vi "IV.vi"(2 "Run uninterrupted?":bool, 3 "Device Category IN:":string(combo)="ATLAS18SS" caption="Device Category:", 4 "Batch No. IN:":string caption="Batch No.:", 5 "Wafer No. IN:":string caption="Wafer No.:", 6 "DB Serial No. IN:":string caption="DB Serial No.:") -> (0 "Done!":bool)   [LabVIEW 2013]
doc: "Performs IV measurements according to ATLAS ITk Quality Control Specifications."
uses:
  InstrControl/Switching/Switching.lvclass
  InstrControl/SupplyControl/SupplyControl.lvclass
  general_VIs/globals/QC_MeasurementSetup.vi
  general_VIs/globals/QC_RunInformation.vi
  InstrControl/InstrumentSetup.vi
  InstrControl/ArduinoControl/ArduinoControl.lvclass
  <vilib>/Analysis/NI_AALBase.lvlib
  InstrControl/InstrControl.lvclass
panel:
  out "Tab Control 2":enum32{"IV Setup", "IV Scan"}(tab)
  in  "V_breakdown limit [V]":dbl=-500.0
  in  "Set current limit?":bool
  in  "Current Limit [µA]":dbl=1000.0 min=0.0001 format="%.3f"
  in  "Measurement Configurations":bool
  in  "hold steps IN":i32=6 caption="hold steps"
  in  "Initial volts [V] IN":dbl caption="Initial volts [V]"
  in  "Final volts [V] IN":dbl=-700.0 caption="Final volts [V]"
  in  "step [V] IN":dbl=10.0 caption="step [V]" format="%.1f"
  in  "step interval [s] IN":i32=10 caption="step interval [s]"
  in  "Continue":bool
  in  "Quit":bool
  out "hold steps":i32=6
  out "RH":dbl[](array[numeric]) caption="RH [%]" format="%#.2f"
  out "Temp.":dbl[](array[numeric]) caption="Temp. [°C]" format="%#.2f"
  out "Current":dbl[](array[numeric]) caption="Current [nA]"
  out "Volts":dbl[](array[numeric]) caption="Volts [V]"
  out "step interval [s]":i32=10
  out "step [V]":dbl=10.0 format="%.1f"
  out "Final volts [V]":dbl=-700.0 format="%.1f"
  out "Initial volts [V]":dbl format="%.1f"
  out "Igraph":cluster{dbl[], dbl[]}(graph)
  in  "Scales":T1(ring)
  in  "Iscale":enum16{"nanoAmps", "microAmps", "milliAmps"}(ring)
  out "positive ramp?":bool
  out "Tab Control":enum32{"IV Setup", "IV Scan"}(tab)
  in  "Hardware Configurations":bool
  in  "User:":string(combo)="Christoph"
  in  "IV Supply":string(combo)="Keithley 2410"
  in  "Temperature":enum16{"Read Arduino", "Enter manually"}(ring)
  in  "Manufacturer:":string(combo)="Hamamatsu"
  in  "abort":bool
  out "Device Category:":string
  out "DB Serial No.:":string
  out "Current Volts:":dbl format="%.2f"
  in  "quit (no save)":bool
  in  "Quit & Save":bool
  out "Bias On/Off:":bool
  out "STATUS 1":string
  out "Initiated:":string
  out "Sensor No.:":string
  out "No of steps":u32
  out "Current reading No.":u32
  out "Last reading at:":string
  # "University of\nCambridge"
  # "Strip Sensor QC: IV"
  # "Vertical Scale:"
  # "Measurement Configuration"
  # "IV Scan parameters:"
  # "Last 5 readings:"
  # "n-4"
  # "n-3"
  # "n-2"
  # "n-1"
  # "n"
  # "DUT Description"
  # "Hardware"
  # "DUT & Test Description:"
  # "Current status:"
  # "Rdg No:"
  # "out of"
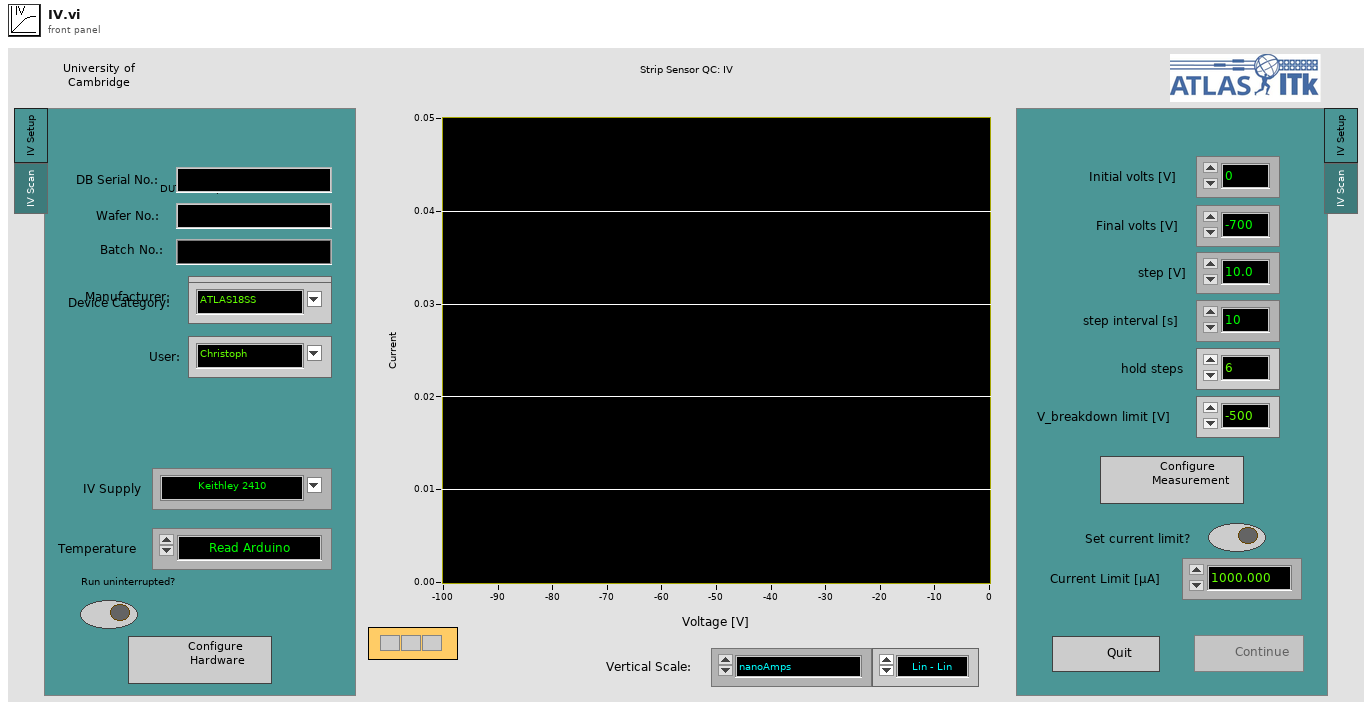
[diagram p1: front panel]
types:
  T1 = enum16{"Lin - Lin", "Log - Lin", "Lin - Log", "Log - log"}
  T2 = enum16{"Supply", "LCR", "Multimeter", "Switching"}
  T3 = enum16{"Reset", "Read Array", "Read Element", "Write Element", "Write Array", "Add Element", "Add Array"}
  T4 = enum16{"Reset", "Ground", "Striptest SMU", "Striptest LCR", "IV", "CV", "Interstrip Cap", "Interstrip Res"}
  T5 = enum32{"IV", "CV", "Stability", "Striptest", "Cis", "Ris", "PTP"}
  T6 = cluster{"Institute":string, "Manufacturers":string[], "Devices":string[], "Serialnumbers Lookup DB":string, "Data directory":string, "Backup & screenshot directory":string, "List of known users":string[], "Measurement switch not used":bool, "Measurement Switch":string, "DUT Switch":string, "Rseries IV [MOhm]":string, "Rshunt IV [MOhm]":string, "Rseries CV [MOhm]":string, "DC blocking Cap [µF]":string, "Rseries LCR [MOhm]":string, "Rseries stability [MOhm]":string, "Rshunt stability [MOhm]":string, "Rseries striptest bias [MOhm]":string, "Rseries strip pinhole [MOhm]":string}
  T7 = cluster{"Sensor Serial No.:":string, "Wafer:":string, "Batch:":string, "Manufacturer:":string, "Device Category:":string, "Database Serial No.:":string, "Date Initiated:":string, "Time Initiated:":string, "Test":string, "Probeplan used:":string, "End of Run comment:":string, "User:":string, "Vbias SMU":string, "LCR":string, "Test SMU":string, "Test DMM":string}
  T8 = cluster{"Supply":refnum<class "SupplyControl.lvclass">, "Arduino":refnum<class "ArduinoControl.lvclass">, "Measurement switch":refnum<class "Switching.lvclass">, "Initial Voltage [V]":dbl, "Final Voltage [V]":dbl, "Step Size [V]":dbl, "Step Interval [s]":i32, "Number Of Steps":u32, "Ramp down steps [V]":dbl, "Ramp down Interval [s]":i32, "hold steps":i32, "Set Current Limit?":bool, "Current Limit [µA]":dbl, "Temperature Readout":enum16{"Read Arduino", "Enter manually"}, "Supply Name":string, "V_breakdown Limit [V]":dbl, "Measurement switch used?":bool}
  T9 = cluster{"VISA address":refnum<visa-resource-name>, "T sensor":enum16{"SHT", "DS"}, "Arduino":refnum<class "ArduinoControl.lvclass">}
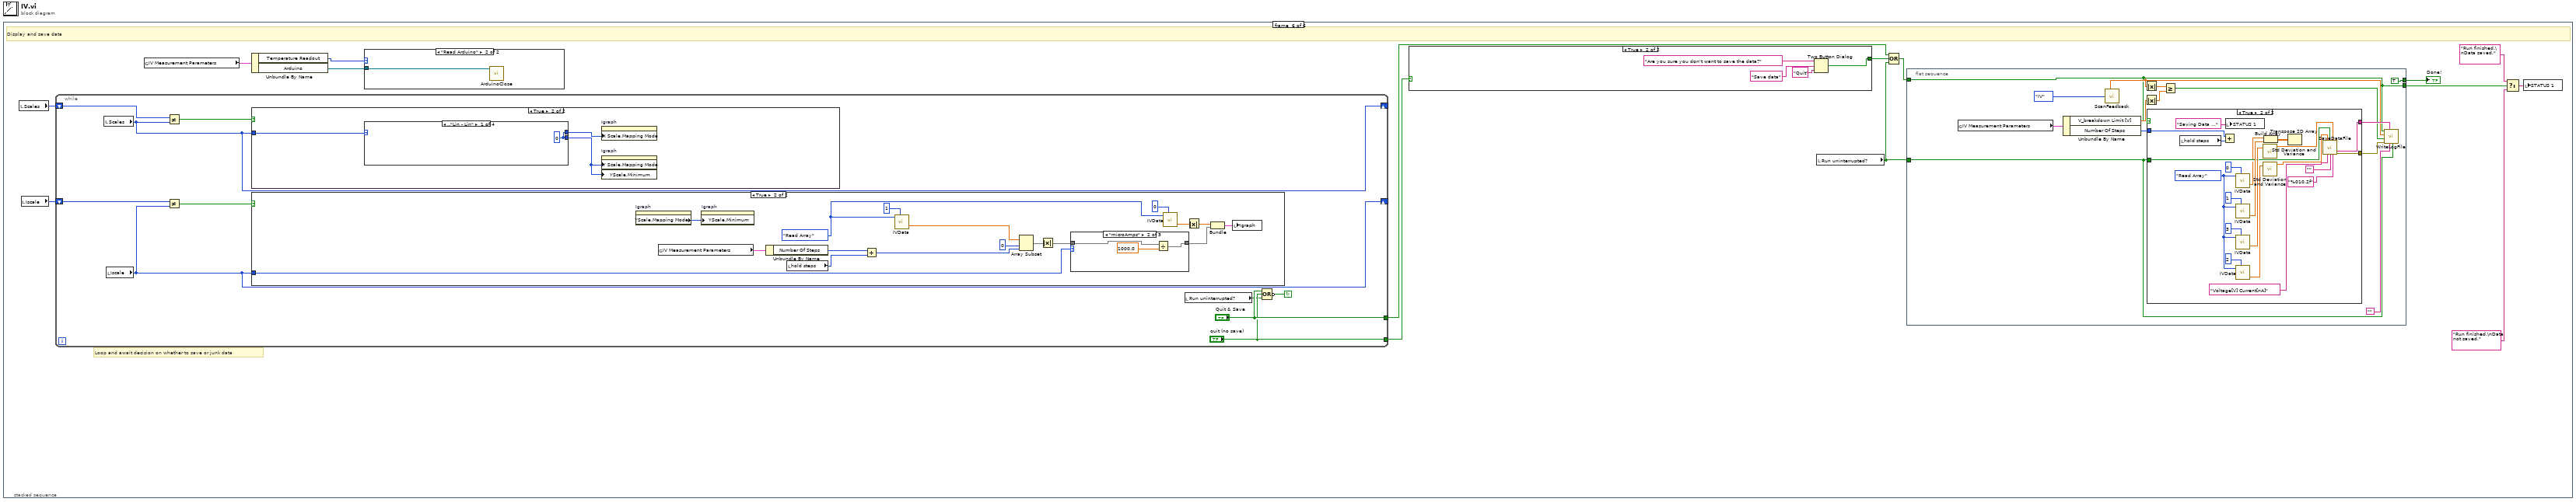
[diagram p0: block diagram]
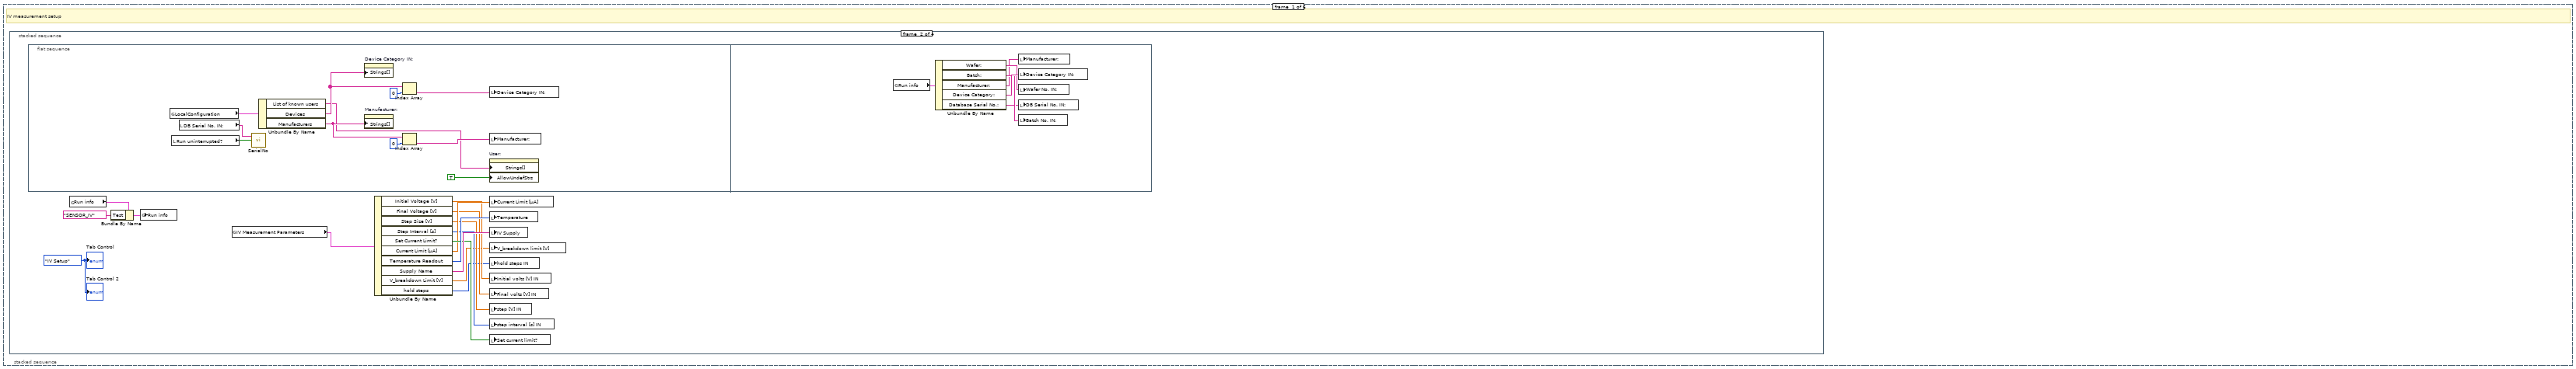
[diagram p2: hidden frame]
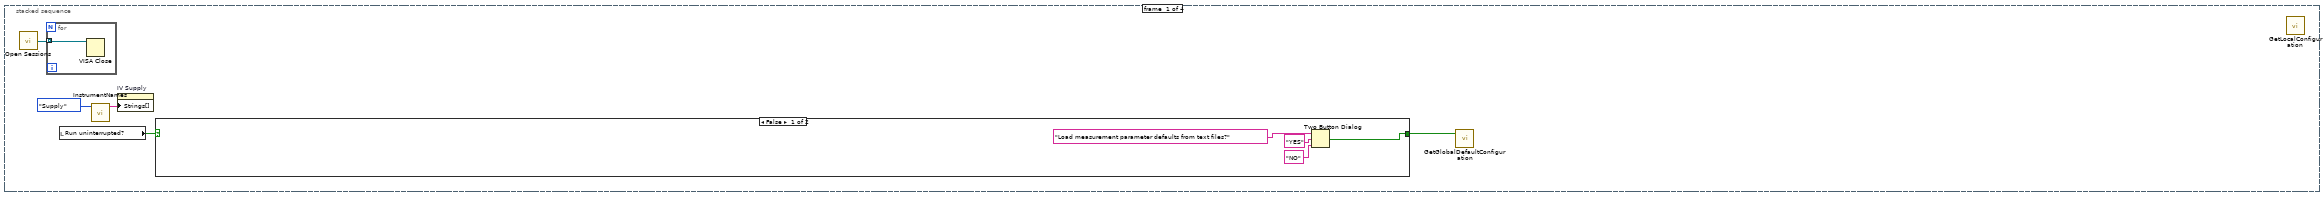
[diagram p3: hidden frame]
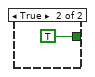
[diagram p4: hidden frame]
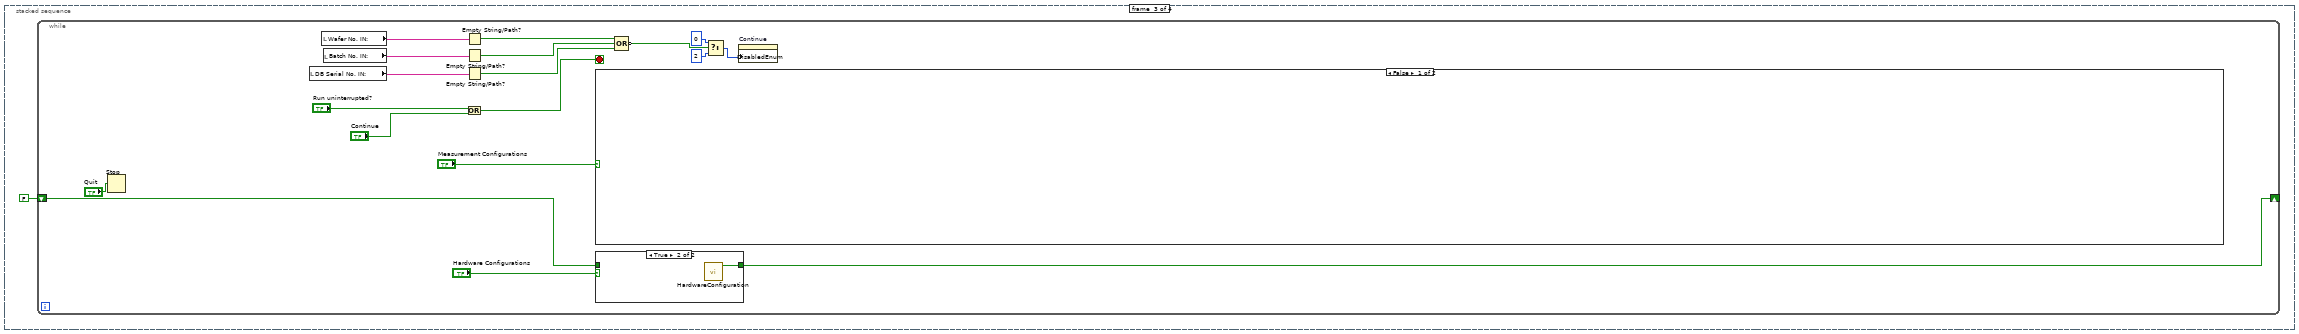
[diagram p5: hidden frame]
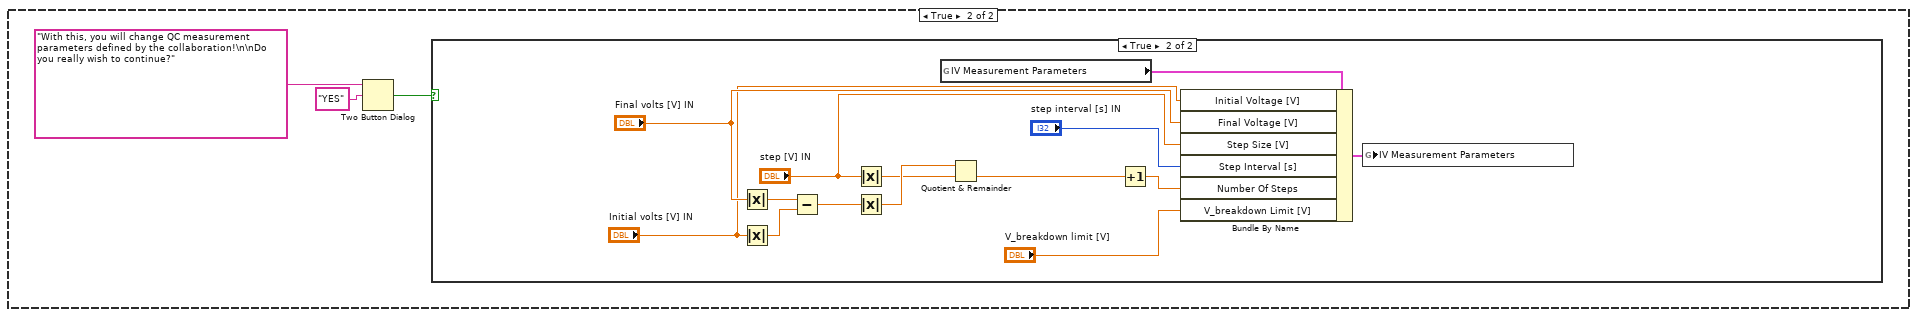
[diagram p6: hidden frame]
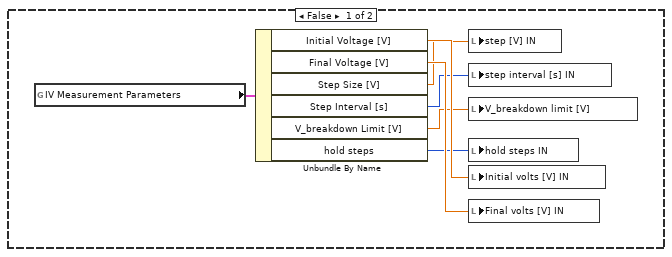
[diagram p7: hidden frame]
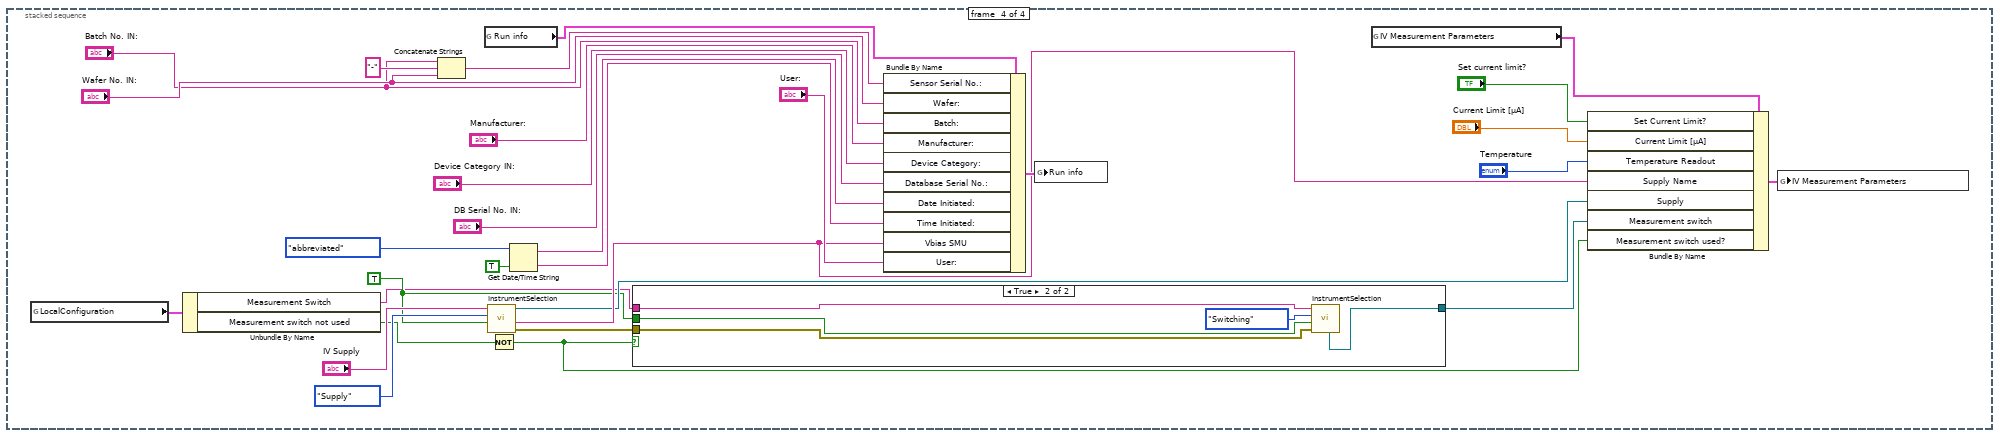
[diagram p9: hidden frame]
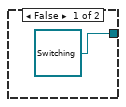
[diagram p10: hidden frame]
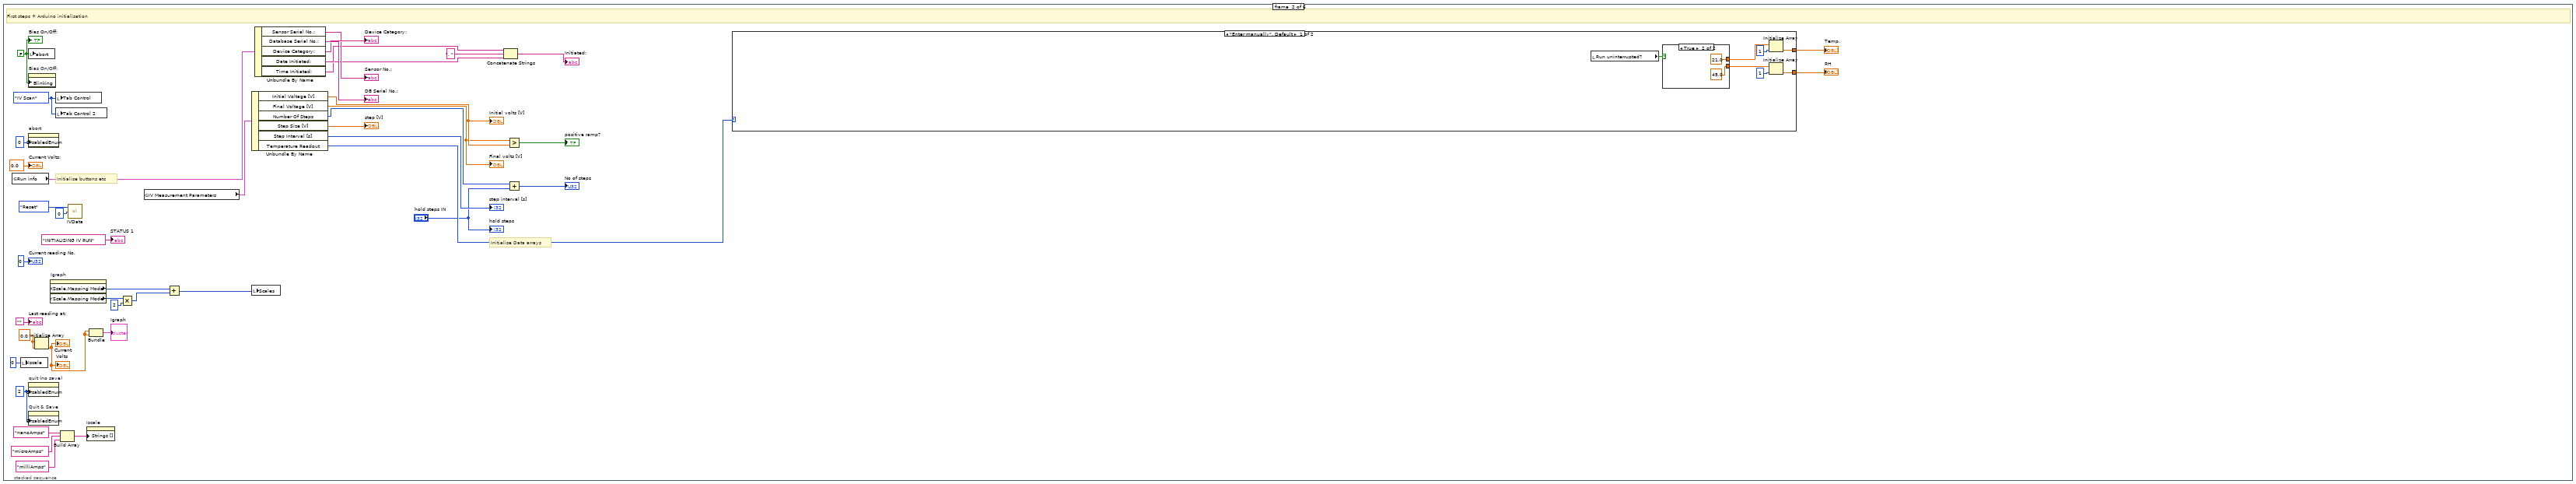
[diagram p11: hidden frame]
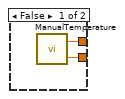
[diagram p12: hidden frame]
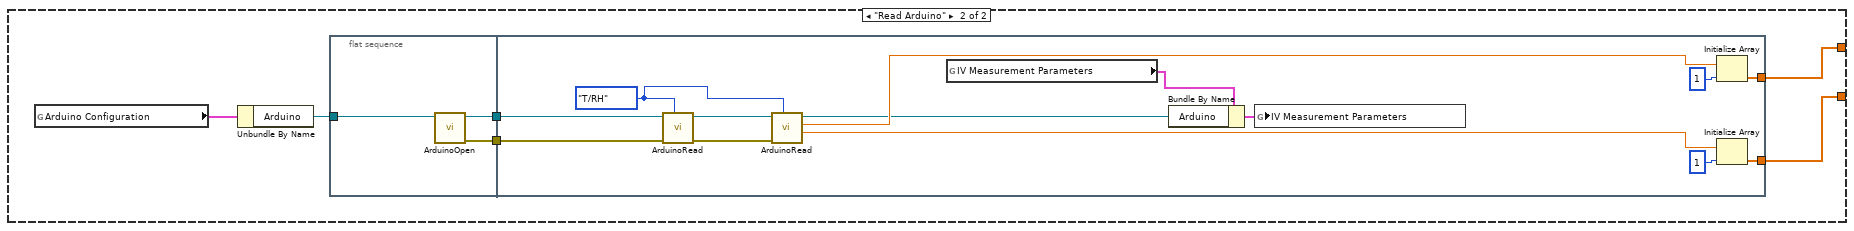
[diagram p13: hidden frame]
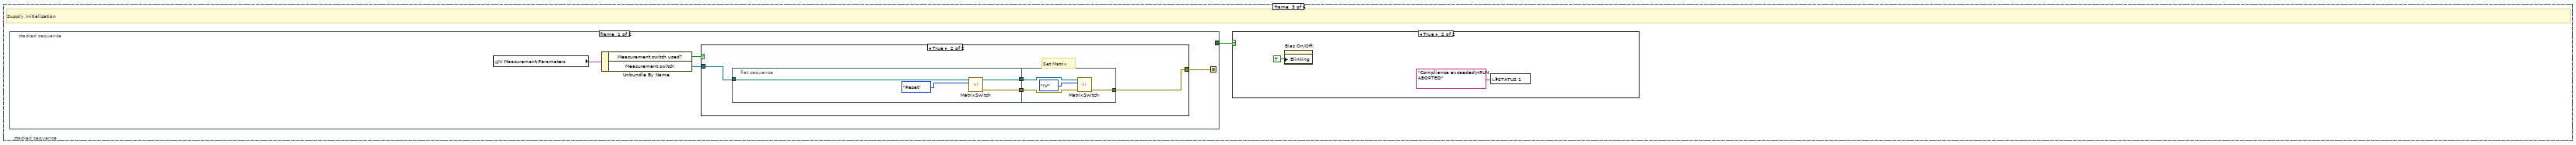
[diagram p14: hidden frame]
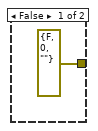
[diagram p15: hidden frame]
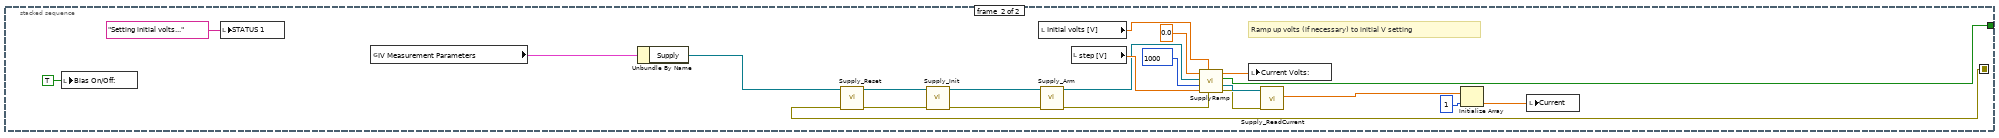
[diagram p16: hidden frame]
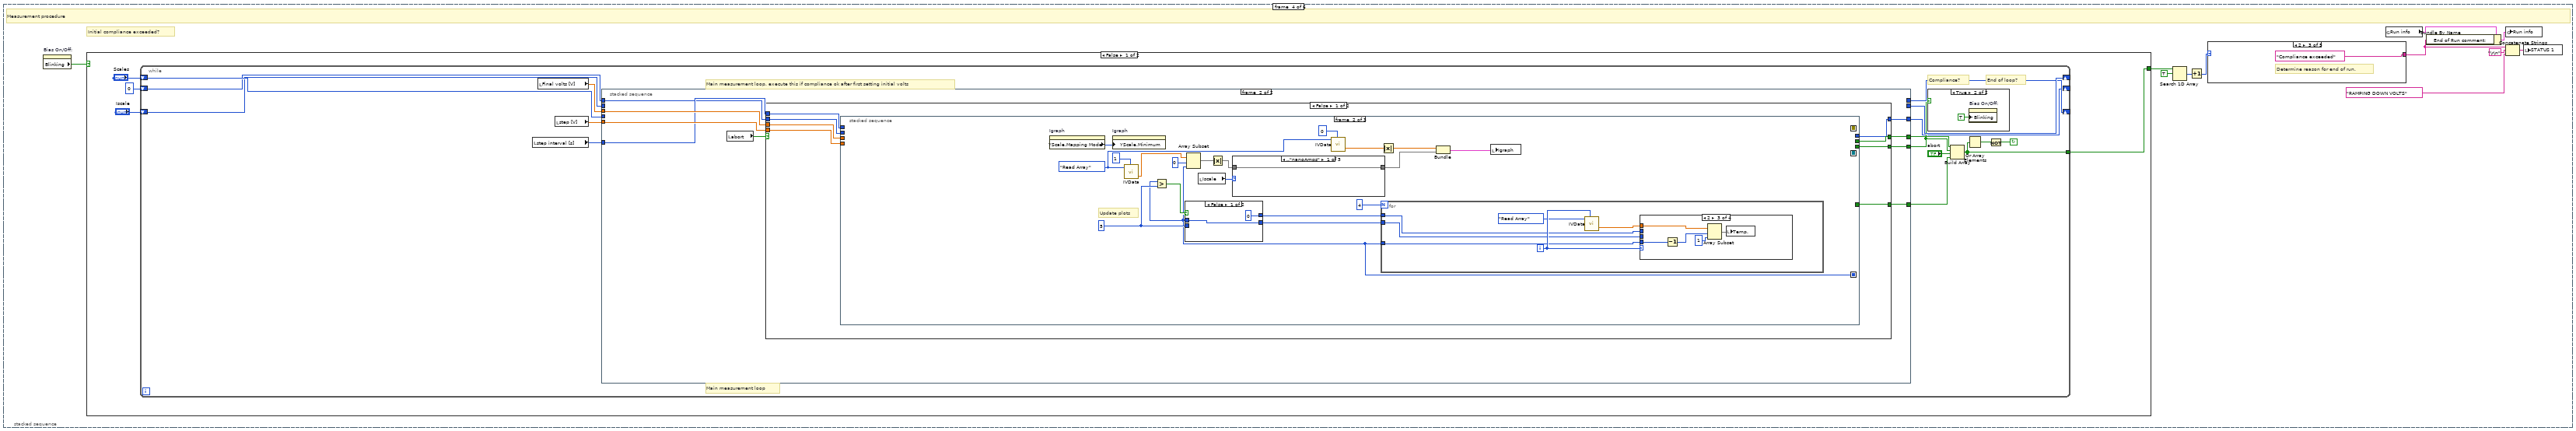
[diagram p18: hidden frame]
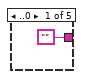
[diagram p19: hidden frame]
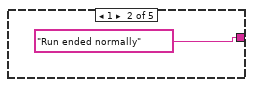
[diagram p20: hidden frame]
diagram:
  n1 = stacked-sequence {
    frame #0 {
      # "IV measurement setup"
      n2 = stacked-sequence {
        frame #0 {
          n3 = call <vilib>:"Open Sessions.vi"() -> ("Array of Refnums"=w1:refnum<visa-resource-name>[])  [unwired: 2 in]
          n4 = for {
            tunnel: w1 -> [w6] mode=indexing
            n5 = VISA Close(VISA resource name=w6) -> ()  [unwired: 1 in, 1 out]
          }
          n6 = local read "Run uninterrupted?"() -> (w2:bool)
          n7 = call "InstrumentNames.vi"("Instrument type"=T2."Supply") -> ("Instrument names"=w4:string[])  [unwired: 9 in, 1 out]
          n8 = property on="IV Supply" class="CmbBox"("Strings[]"=w4) -> ()  [unwired: 2 in, 2 out]
          n9 = case shown="False" w2 {
            tunnel: [w9 TRUE] -> w3
            frame False {
              n10 = Two Button Dialog(message="Load measurement parameter defaults from text files?", 1:"NO", 2:"YES") -> (T button?=w9:bool)
            }
            frame True {
            }
          }
          n11 = call "GetGlobalDefaultConfiguration.vi"("Read defaults?"=w3) -> ()  [unwired: 3 in]
          n12 = call "GetLocalConfiguration.vi"() -> ()  [unwired: 3 in, 1 out]
        }
        frame #1 {
          w19 = enum32{"IV Setup", "IV Scan"}."IV Setup" ("Tab Control")
          n13 = flat-sequence {
            frame #0 {
              n14 = global read "QC_RunInformation.vi" "LocalConfiguration"() -> (w29:T6)
              n15 = local read "Run uninterrupted?"() -> (w28:bool)
              n16 = local read "DB Serial No. IN:"() -> (w27:string)
              n17 = call "SerialNo.vi"("DB serial number IN"=w27, "Run uninterrupted?"=w28) -> ()  [unwired: 6 in, 2 out]
              n18 = Unbundle By Name(w29) -> ("List of known users"=w30:string[], "Devices"=w33:string[], "Manufacturers"=w35:string[])
              n19 = property on="Device Category IN:" class="CmbBox"("Strings[]"=w33) -> ()  [unwired: 2 in, 2 out]
              n20 = property on="Manufacturer:" class="CmbBox"("Strings[]"=w35) -> ()  [unwired: 2 in, 2 out]
              n21 = Index Array(array=w33, index=0) -> (element=w37:string)
              n22 = Index Array(array=w35, index=0) -> (element=w36:string)
              n23 = local write "Device Category IN:"(w37) -> ()
              n24 = local write "Manufacturer:"(w36) -> ()
              n25 = property on="User:" class="CmbBox"("Strings[]"=w30, "AllowUndefStrs"=TRUE) -> ()  [unwired: 2 in, 2 out]
            }
            frame #1 {
              n26 = global read "QC_RunInformation.vi" "Run info"() -> (w38:T7)
              n27 = Unbundle By Name(w38) -> ("Wafer:"=w42:string, "Batch:"=w41:string, "Manufacturer:"=w40:string, "Device Category:"=w43:string, "Database Serial No.:"=w39:string)
              n28 = local write "Manufacturer:"(w40) -> ()
              n29 = local write "Device Category IN:"(w43) -> ()
              n30 = local write "Wafer No. IN:"(w42) -> ()
              n31 = local write "DB Serial No. IN:"(w39) -> ()
              n32 = local write "Batch No. IN:"(w41) -> ()
            }
          }
          n33 = global read "QC_RunInformation.vi" "Run info"() -> (w21:T7)
          n34 = Bundle By Name(cluster=w21, "Test"="SENSOR_IV") -> (w20:T7)
          n35 = global write "QC_RunInformation.vi" "Run info"(w20) -> ()
          n36 = global read "QC_MeasurementSetup.vi" "IV Measurement Parameters"() -> (w24:T8)
          n37 = Unbundle By Name(w24) -> ("Initial Voltage [V]"=w17:dbl, "Final Voltage [V]"=w16:dbl, "Step Size [V]"=w15:dbl, "Step Interval [s]"=w18:i32, "Set Current Limit?"=w23:bool, "Current Limit [µA]"=w22:dbl, "Temperature Readout"=w26:enum16{"Read Arduino", "Enter manually"}, "Supply Name"=w25:string, "V_breakdown Limit [V]"=w14:dbl, "hold steps"=w13:i32)
          n38 = local write "Current Limit [µA]"(w22) -> ()
          n39 = local write "Temperature"(w26) -> ()
          n40 = local write "IV Supply"(w25) -> ()
          n41 = local write "V_breakdown limit [V]"(w14) -> ()
          n42 = local write "hold steps IN"(w13) -> ()
          n43 = local write "Initial volts [V] IN"(w17) -> ()
          n44 = local write "Final volts [V] IN"(w16) -> ()
          n45 = local write "step [V] IN"(w15) -> ()
          n46 = local write "step interval [s] IN"(w18) -> ()
          n47 = local write "Set current limit?"(w23) -> ()
          "Tab Control" <- w19
          "Tab Control 2" <- w19
        }
        frame #2 {
          n48 = while {
            shift-right: [w52] -> _
            shift-left: FALSE -> [w51]
            stop <- w48 stop-if-true
            n49 = Stop(stop? (T)="Quit") -> ()
            n50 = local read "DB Serial No. IN:"() -> (w46:string)
            n51 = local read "Wafer No. IN:"() -> (w61:string)
            n52 = local read "Batch No. IN:"() -> (w54:string)
            n53 = Empty String/Path?(string/path=w61) -> (empty?=w60:bool)
            n54 = Empty String/Path?(string/path=w54) -> (empty?=w53:bool)
            n55 = Empty String/Path?(string/path=w46) -> (empty?=w45:bool)
            n56 = Or(x="Run uninterrupted?", y="Continue") -> (x .or. y?=w48:bool)
            n57 = case shown="False" "Measurement Configurations" {
              frame False {
              }
              frame True {
                n58 = Two Button Dialog(message="With this, you will change QC measurement parameters defined by the collaboration!\n\nDo you really wish to continue?", 2:"YES") -> (T button?=w63:bool)  [unwired: 1 in]
                n59 = case shown="True" w63 {
                  frame False {
                    n60 = global read "QC_MeasurementSetup.vi" "IV Measurement Parameters"() -> (w72:T8)
                    n61 = Unbundle By Name(w72) -> ("Initial Voltage [V]"=w70:dbl, "Final Voltage [V]"=w71:dbl, "Step Size [V]"=w69:dbl, "Step Interval [s]"=w68:i32, "V_breakdown Limit [V]"=w67:dbl, "hold steps"=w66:i32)
                    n62 = local write "step [V] IN"(w69) -> ()
                    n63 = local write "step interval [s] IN"(w68) -> ()
                    n64 = local write "V_breakdown limit [V]"(w67) -> ()
                    n65 = local write "hold steps IN"(w66) -> ()
                    n66 = local write "Initial volts [V] IN"(w70) -> ()
                    n67 = local write "Final volts [V] IN"(w71) -> ()
                  }
                  frame True {
                    n68 = Absolute Value(x="Final volts [V] IN") -> (abs(x)=w82:dbl)
                    n69 = Absolute Value(x="Initial volts [V] IN") -> (abs(x)=w81:dbl)
                    n70 = Subtract(x=w82, y=w81) -> (x-y=w76:dbl)
                    n71 = Absolute Value(x="step [V] IN") -> (abs(x)=w77:dbl)
                    n72 = Absolute Value(x=w76) -> (abs(x)=w78:dbl)
                    n73 = global read "QC_MeasurementSetup.vi" "IV Measurement Parameters"() -> (w86:T8)
                    n74 = Quotient & Remainder(x=w78, y=w77) -> (floor(x/y)=w74:dbl)  [unwired: 1 out]
                    n75 = Increment(x=w74) -> (x+1=w73:dbl)
                    n76 = Bundle By Name(cluster=w86, "Initial Voltage [V]"="Initial volts [V] IN", "Final Voltage [V]"="Final volts [V] IN", "Step Size [V]"="step [V] IN", "Step Interval [s]"="step interval [s] IN", "Number Of Steps"=w73, "V_breakdown Limit [V]"="V_breakdown limit [V]") -> (w83:T8)
                    n77 = global write "QC_MeasurementSetup.vi" "IV Measurement Parameters"(w83) -> ()
                  }
                }
              }
            }
            n78 = case shown="True" "Hardware Configurations" {
              tunnel: [w87 w88] -> w52
              tunnel: w51 -> [w87 _]
              frame False {
              }
              frame True {
                n79 = call "HardwareConfiguration.vi"() -> ("configured?"=w88:bool)  [unwired: 11 in]
              }
            }
            n80 = Compound Arithmetic op=OR(w60, w53, w45) -> (invert w59:bool)
            n81 = Select(t=0, s=w59, f=2) -> (s? t:f=w56:i32)
            n82 = property on="Continue" class="Bool"("DisabledEnum"=w56) -> ()  [unwired: 2 in, 2 out]
          }
        }
        frame #3 {
          w102 = TRUE
          n83 = global read "QC_RunInformation.vi" "LocalConfiguration"() -> (w92:T6)
          n84 = Unbundle By Name(w92) -> ("Measurement Switch"=w90:string, "Measurement switch not used"=w91:bool)
          n85 = Concatenate Strings("Batch No. IN:", "-", "Wafer No. IN:") -> (w94:string)
          n86 = global read "QC_RunInformation.vi" "Run info"() -> (w93:T7)
          n87 = call "InstrumentSelection.vi"("Verify GPIB address"=w102, "Instrument type"=T2."Supply", "Instrument name IN"="IV Supply") -> ("error out"=w104:errorcluster, "Instrument name OUT"=w106:string, "Supply"=w105:refnum<class "SupplyControl.lvclass">)  [unwired: 3 in, 3 out]
          n88 = Not(x=w91) -> (.not. x?=w89:bool)
          n89 = Get Date/Time String(date format (0)=enum16{"short", "long", "abbreviated"}."abbreviated", want seconds? (F)=TRUE) -> (date string=w99:string, time string=w98:string)  [unwired: 1 in]
          n90 = case shown="True" w89 {
            tunnel: w104 -> [_ w123]
            tunnel: [refnum<class "Switching.lvclass"> refnum ("Switching") w122] -> w103
            tunnel: w102 -> [_ w121]
            tunnel: w90 -> [_ w120]
            frame False {
            }
            frame True {
              n91 = call "InstrumentSelection.vi"("error in (no error)"=w123, "Verify GPIB address"=w121, "Instrument type"=T2."Switching", "Instrument name IN"=w120) -> ("Switching"=w122:refnum<class "Switching.lvclass">)  [unwired: 2 in, 5 out]
            }
          }
          n92 = Bundle By Name(cluster=w93, "Sensor Serial No.:"=w94, "Wafer:"="Wafer No. IN:", "Batch:"="Batch No. IN:", "Manufacturer:"="Manufacturer:", "Device Category:"="Device Category IN:", "Database Serial No.:"="DB Serial No. IN:", "Date Initiated:"=w99, "Time Initiated:"=w98, "Vbias SMU"=w106, "User:"="User:") -> (w112:T7)
          n93 = global write "QC_RunInformation.vi" "Run info"(w112) -> ()
          n94 = global read "QC_MeasurementSetup.vi" "IV Measurement Parameters"() -> (w117:T8)
          n95 = Bundle By Name(cluster=w117, "Set Current Limit?"="Set current limit?", "Current Limit [µA]"="Current Limit [µA]", "Temperature Readout"="Temperature", "Supply Name"=w106, "Supply"=w105, "Measurement switch"=w103, "Measurement switch used?"=w89) -> (w118:T8)
          n96 = global write "QC_MeasurementSetup.vi" "IV Measurement Parameters"(w118) -> ()
        }
      }
    }
    frame #1 {
      w132 = enum32{"IV Setup", "IV Scan"}."IV Scan" ("Tab Control")
      w150 = 2
      w157 = 0.0
      w149 = FALSE ("Visible")
      # "Initialise buttons etc"
      # "Initialise Data arrays"
      # "First steps + Arduino initialisation"
      n97 = global read "QC_RunInformation.vi" "Run info"() -> (w166:T7)
      n98 = local write "Iscale"(u16 0 ("Scale")) -> ()
      n99 = local write "abort"(w149) -> ()
      n100 = property on="Bias On/Off:" class="Bool (strict)"("Blinking"=w149) -> ()  [unwired: 2 in, 2 out]
      n101 = property on="abort" class="Bool (strict)"("DisabledEnum"=0) -> ()  [unwired: 2 in, 2 out]
      n102 = property on="quit (no save)" class="Bool"("DisabledEnum"=w150) -> ()  [unwired: 2 in, 2 out]
      n103 = property on="Quit & Save" class="Bool"("DisabledEnum"=w150) -> ()  [unwired: 2 in, 2 out]
      n104 = Initialize Array(w157, w157) -> (w134:dbl[])
      "Volts" <- w134
      "Current" <- w134
      n105 = property on="Igraph" class="XYGraph (strict)"() -> ("XScale.Mapping Mode"=w143:u8, "YScale.Mapping Mode"=w142:u8)  [unwired: 2 in, 2 out]
      n106 = local write "Tab Control"(w132) -> ()
      n107 = local write "Tab Control 2"(w132) -> ()
      n108 = Build Array("nanoAmps", "microAmps", "milliAmps") -> (w163:string[])
      n109 = call "IVData.vi"("Action"=T3."Reset", "Array Size / Index"=0) -> ()  [unwired: 3 in, 2 out]
      n110 = property on="Iscale" class="Enum (strict)"("Strings []"=w163) -> ()  [unwired: 2 in, 2 out]
      n111 = Bundle(w134, w134) -> (→"Igraph":cluster{dbl[], dbl[]})  [unwired: 1 in]
      n112 = Multiply(x=w142, y=2) -> (x*y=w145:i32)
      n113 = global read "QC_MeasurementSetup.vi" "IV Measurement Parameters"() -> (w139:T8)
      n114 = Add(x=w143, y=w145) -> (x+y=w141:i32)
      n115 = Unbundle By Name(w139) -> ("Initial Voltage [V]"=w148:dbl, "Final Voltage [V]"=w147:dbl, "Number Of Steps"=w136:u32, "Step Size [V]"=→"step [V]":dbl, "Step Interval [s]"=→"step interval [s]":i32, "Temperature Readout"=w151:enum16{"Read Arduino", "Enter manually"})
      "Initial volts [V]" <- w148
      "Final volts [V]" <- w147
      n116 = local write "Scales"(w141) -> ()
      n117 = Unbundle By Name(w166) -> ("Sensor Serial No.:"=→"Sensor No.:":string, "Database Serial No.:"=→"DB Serial No.:":string, "Device Category:"=→"Device Category:":string, "Date Initiated:"=w130:string, "Time Initiated:"=w129:string)
      n118 = Concatenate Strings(w130, ", ", w129) -> (→"Initiated:":string)
      n119 = Greater?(x=w147, y=w148) -> (0:→"positive ramp?":bool)
      n120 = Add(x=w136, y="hold steps IN") -> (x+y=→"No of steps":u32)
      n121 = case shown="\"Enter manually\", Default" w151 {
        tunnel: [w174 w184] -> w154
        tunnel: [w173 w183] -> w140
        frame "Enter manually", Default {
          n122 = local read "Run uninterrupted?"() -> (w168:bool)
          n123 = case shown="True" w168 {
            tunnel: [w176 21.0] -> w172
            tunnel: [w175 45.0] -> w169
            frame False {
              n124 = call "ManualTemperature.vi"() -> ("Humidity [%] out"=w175:dbl, "Temperature [°C] out"=w176:dbl)
            }
            frame True {
            }
          }
          n125 = Initialize Array(w172, 1) -> (w174:dbl[])
          n126 = Initialize Array(w169, 1) -> (w173:dbl[])
        }
        frame "Read Arduino" {
          n127 = global read "InstrumentSetup.vi" "Arduino Configuration"() -> (w180:T9)
          n128 = Unbundle By Name(w180) -> ("Arduino"=w179:refnum<class "ArduinoControl.lvclass">)
          n129 = flat-sequence {
            tunnel: [w185] -> w182
            tunnel: [w187] -> w181
            tunnel: w179 -> [w186]
            tunnel: [w201] -> w184
            tunnel: [w198] -> w183
            tunnel: w182 -> [w192]
            tunnel: w181 -> [w191]
            frame #0 {
              n130 = call "ArduinoOpen.vi"("ArduinoControl in"=w186) -> ("error out"=w187:errorcluster, "ArduinoControl out"=w185:refnum<class "ArduinoControl.lvclass">)  [unwired: 9 in]
            }
            frame #1 {
              w188 = enum16{"T/RH", "Interlock", "Edgesense"}."T/RH" ("Arduino function")
              n131 = call "ArduinoRead.vi"("Arduino function"=w188, "error in (no error)"=w191, "ArduinoControl in"=w192) -> ("error out"=w190:errorcluster, "ArduinoControl out"=w189:refnum<class "ArduinoControl.lvclass">)  [unwired: 3 in, 4 out]
              n132 = call "ArduinoRead.vi"("Arduino function"=w188, "error in (no error)"=w190, "ArduinoControl in"=w189) -> ("rel. Humidity [%]"=w196:dbl, "Temperature [°C]"=w197:dbl, "ArduinoControl out"=w195:refnum<class "ArduinoControl.lvclass">)  [unwired: 3 in, 3 out]
              n133 = global read "QC_MeasurementSetup.vi" "IV Measurement Parameters"() -> (w194:T8)
              n134 = Bundle By Name(cluster=w194, "Arduino"=w195) -> (w193:T8)
              n135 = global write "QC_MeasurementSetup.vi" "IV Measurement Parameters"(w193) -> ()
              n136 = Initialize Array(w197, 1) -> (w201:dbl[])
              n137 = Initialize Array(w196, 1) -> (w198:dbl[])
            }
          }
        }
      }
      "Temp." <- w154
      "RH" <- w140
      "STATUS 1" <- "INITIALISING IV RUN"
      "Bias On/Off:" <- w149
      "Last reading at:" <- ""
      "Current reading No." <- u32 0 ("Current reading No.")
      "Current Volts:" <- 0.0 ("Current Volts:")
      "hold steps" <- "hold steps IN"
    }
    frame #2 {
      # "Supply initialisation"
      n138 = stacked-sequence {
        seq-local: [w204 _] -> [_ w220]
        tunnel: [_ w221] -> w202
        frame #0 {
          n139 = global read "QC_MeasurementSetup.vi" "IV Measurement Parameters"() -> (w203:T8)
          n140 = Unbundle By Name(w203) -> ("Measurement switch used?"=w206:bool, "Measurement switch"=w205:refnum<class "Switching.lvclass">)
          n141 = case shown="True" w206 {
            tunnel: w205 -> [_ w208]
            tunnel: [errorcluster {"status"=FALSE, "code"=0, "source"=""} ("error constant") w209] -> w204
            frame False {
            }
            frame True {
              # "Set Matrix"
              n142 = flat-sequence {
                tunnel: [w215] -> w211
                tunnel: [w214] -> w210
                tunnel: w208 -> [w212]
                tunnel: w211 -> [w219]
                tunnel: w210 -> [w218]
                tunnel: [w217] -> w209
                frame #0 {
                  n143 = call-dynamic "MatrixSwitch.vi"("Action"=T4."Reset", "Switching in"=w212) -> ("error out"=w215:errorcluster, "Switching out"=w214:refnum<class "Switching.lvclass">)  [unwired: 7 in, 1 out]
                }
                frame #1 {
                  n144 = call-dynamic "MatrixSwitch.vi"("error in (no error)"=w219, "Action"=T4."IV", "Switching in"=w218) -> ("error out"=w217:errorcluster)  [unwired: 6 in, 2 out]
                }
              }
            }
          }
        }
        frame #1 {
          # "Ramp up volts (if necessary) to initial V setting"
          n145 = local write "Bias On/Off:"(TRUE ("Compliance?")) -> ()
          n146 = local write "STATUS 1"("Setting initial volts..." ("STATUS 1")) -> ()
          n147 = global read "QC_MeasurementSetup.vi" "IV Measurement Parameters"() -> (w237:T8)
          n148 = Unbundle By Name(w237) -> ("Supply"=w234:refnum<class "SupplyControl.lvclass">)
          n149 = call-dynamic "Supply_Reset.vi"("error in (no error)"=w220, "SupplyControl in"=w234) -> ("error out"=w239:errorcluster, "SupplyControl out"=w241:refnum<class "SupplyControl.lvclass">)  [unwired: 8 in]
          n150 = call-dynamic "Supply_Init.vi"("error in (no error)"=w239, "SupplyControl in"=w241) -> ("error out"=w238:errorcluster, "SupplyControl out"=w240:refnum<class "SupplyControl.lvclass">)  [unwired: 8 in]
          n151 = local read "Initial volts [V]"() -> (w229:dbl)
          n152 = call-dynamic "Supply_Arm.vi"("error in (no error)"=w238, "SupplyControl in"=w240) -> ("error out"=w227:errorcluster, "SupplyControl out"=w228:refnum<class "SupplyControl.lvclass">)  [unwired: 8 in]
          n153 = local read "step [V]"() -> (w230:dbl)
          n154 = call "SupplyRamp.vi"("error in"=w227, "Requested Voltage"=w229, "Step Size"=w230, "Step Delay"=1000, "Supply IN"=w228, "Starting Voltage"=0.0) -> ("error out"=w222:errorcluster, "Supply OUT"=w223:refnum<class "SupplyControl.lvclass">, "Compliance exceeded"=w221:bool, "Current Voltage"=w233:dbl)  [unwired: 2 in]
          n155 = local write "Current Volts:"(w233) -> ()
          n156 = call-dynamic "Supply_ReadCurrent.vi"("error in (no error)"=w222, "SupplyControl in"=w223) -> ("Current in nA"=w225:dbl)  [unwired: 7 in, 2 out]
          n157 = Initialize Array(w225, 1) -> (w224:dbl[])
          n158 = local write "Current"(w224) -> ()
        }
      }
      n159 = case shown="True" w202 {
        frame False {
        }
        frame True {
          n160 = property on="Bias On/Off:" class="Bool (strict)"("Blinking"=TRUE) -> ()  [unwired: 2 in, 2 out]
          n161 = local write "STATUS 1"("Compliance exceeded\nRUN ABORTED") -> ()
        }
      }
    }
    frame #3 {
      # "Initial compliance exceeded?"
      # "Measurement procedure"
      n162 = property on="Bias On/Off:" class="Bool (strict)"() -> ("Blinking"=w254:bool)  [unwired: 2 in, 2 out]
      n163 = case shown="False" w254 {
        tunnel: [w263 w508] -> w253
        frame False {
          n164 = while {
            shift-left: "Iscale" -> [w275]
            shift-right: [w274] -> _
            shift-left: "Scales" -> [w276]
            shift-right: [w277] -> _
            tunnel: [w273] -> w263
            shift-right: [w265] -> _
            shift-left: 0 -> [w266]
            stop <- w278 continue-if-true
            # "Main measurement loop"
            # "End of loop?"
            # "Compliance?"
            # "Main measurement loop. execute this if compliance ok after first setting initial volts"
            n165 = local read "step interval [s]"() -> (w270:i32)
            n166 = local read "Final volts [V]"() -> (w271:dbl)
            n167 = local read "step [V]"() -> (w272:dbl)
            n168 = stacked-sequence {
              tunnel: [w292 _] -> w277
              tunnel: w272 -> [w289 w356]
              tunnel: [_ w355] -> w268
              tunnel: w271 -> [_ w354]
              tunnel: w270 -> [w280 w353]
              tunnel: [_ w352] -> w269
              tunnel: w276 -> [w291 _]
              tunnel: w275 -> [w290 _]
              tunnel: [w288 _] -> w274
              tunnel: [_ w350] -> w264
              tunnel: w266 -> [_ w349]
              tunnel: [_ w348] -> w265
              frame #0 {
                n169 = Format Into String(format string="%d", w280) -> (resulting string=w285:string)  [unwired: 2 in, 1 out]
                n170 = Get Date/Time In Seconds() -> (seconds since 1Jan1904=w282:timestamp)
                n171 = To Double Precision Float(number=w282) -> (double precision float=w283:dbl)
                n172 = Concatenate Strings("Waiting for  ", w285, " seconds...") -> (w281:string)
                n173 = while {
                  tunnel: w289 -> [w301]
                  shift-left: w290 -> [w305]
                  shift-right: [w298] -> w288
                  shift-left: w291 -> [w306]
                  shift-right: [w307] -> w292
                  tunnel: w281 -> [w299]
                  tunnel: w280 -> [w311]
                  tunnel: w283 -> [w312]
                  stop <- w313 continue-if-true
                  n174 = Absolute Value(x=w301) -> (abs(x)=w300:dbl)
                  n175 = Get Date/Time In Seconds() -> (seconds since 1Jan1904=w297:timestamp)
                  n176 = local read "Scales"() -> (w307:T1)
                  n177 = local read "Iscale"() -> (w298:enum16{"nanoAmps", "microAmps", "milliAmps"})
                  n178 = Wait (ms)(milliseconds to wait=u32 100) -> ()  [unwired: 1 out]
                  n179 = To Double Precision Float(number=w297) -> (double precision float=w317:dbl)
                  n180 = Not Equal?(x=w305, y=w298) -> (x != y?=w296:bool)
                  n181 = Not Equal?(x=w306, y=w307) -> (x != y?=w308:bool)
                  n182 = Subtract(x=w317, y=w312) -> (x-y=w294:dbl)
                  n183 = local read "abort"() -> (w310:bool)
                  n184 = case shown="True" w296 {
                    tunnel: w300 -> [_ _]
                    tunnel: w298 -> [_ w326]
                    frame False {
                    }
                    frame True {
                      w320 = T3."Read Array" ("Action")
                      n185 = local read "Current reading No."() -> (w328:u32)
                      n186 = property on="Igraph" class="XYGraph (strict)"() -> ("YScale.Mapping Mode"=w322:u8)  [unwired: 2 in, 2 out]
                      n187 = call "IVData.vi"("Action"=w320, "Array No."=u32 1 ("Action")) -> ("Array OUT"=w329:dbl[])  [unwired: 3 in, 1 out]
                      n188 = property on="Igraph" class="XYGraph (strict)"("YScale.Minimum"=w322) -> ()  [unwired: 2 in, 2 out]
                      n189 = Array Subset(array=w329, index=0, length=w328) -> (w325:dbl[])
                      n190 = Absolute Value(x=w325) -> (abs(x)=w324:dbl[])
                      n191 = case shown="\"microAmps\"" w326 {
                        tunnel: [w332 w333 w337] -> w331
                        tunnel: w324 -> [w332 w335 w338]
                        frame .."nanoAmps" {
                        }
                        frame "microAmps" {
                          n192 = Divide(x=w335, y=1000.0) -> (x/y=w333:dbl[])
                        }
                        frame "milliAmps".. {
                          n193 = Divide(x=w338, y=1000000.0) -> (x/y=w337:dbl[])
                        }
                      }
                      n194 = call "IVData.vi"("Action"=w320, "Array No."=u32 0 ("Action")) -> ("Array OUT"=w319:dbl[])  [unwired: 3 in, 1 out]
                      n195 = Absolute Value(x=w319) -> (abs(x)=w318:dbl[])
                      n196 = Bundle(w318, w331) -> (w327:cluster{dbl[], dbl[]})  [unwired: 1 in]
                      n197 = local write "Igraph"(w327) -> ()
                    }
                  }
                  n198 = case shown="True" w308 {
                    tunnel: w307 -> [_ w341]
                    frame False {
                    }
                    frame True {
                      n199 = case shown="\"Log - log\".." w341 {
                        tunnel: [w342 1 0 w347] -> w340
                        tunnel: [w342 0 1 w347] -> w339
                        frame .."Lin - Lin" {
                          w342 = 0
                        }
                        frame "Log - Lin" {
                        }
                        frame "Lin - Log" {
                        }
                        frame "Log - log".. {
                          w347 = 1
                        }
                      }
                      n200 = property on="Igraph" class="XYGraph (strict)"("X Scale.Mapping Mode"=w340) -> ()  [unwired: 2 in, 2 out]
                      n201 = property on="Igraph" class="XYGraph (strict)"("Y Scale.Mapping Mode"=w339, "YScale.Minimum"=w339) -> ()  [unwired: 2 in, 2 out]
                    }
                  }
                  n202 = Subtract(x=w311, y=w294) -> (x-y=w293:dbl)
                  n203 = Format Into String(format string="%d", w293) -> (resulting string=w315:string)  [unwired: 2 in, 1 out]
                  n204 = Not(x=w310) -> (.not. x?=w316:bool)
                  n205 = Greater Than 0?(x=w293) -> (x > 0?=w295:bool)
                  n206 = And(x=w295, y=w316) -> (x .and. y?=w313:bool)
                  n207 = Concatenate Strings(w299, "\r\n", "Timer status: ", w315) -> (w309:string)
                  n208 = local write "STATUS 1"(w309) -> ()
                }
              }
              frame #1 {
                n209 = local read "abort"() -> (w351:bool)
                n210 = case shown="False" w351 {
                  tunnel: [w364 w505] -> w352
                  tunnel: w353 -> [w363 _]
                  tunnel: w354 -> [w362 _]
                  tunnel: [w360 w505] -> w355
                  tunnel: w356 -> [w361 _]
                  tunnel: [w359 w505] -> w350
                  tunnel: w349 -> [w358 w504]
                  tunnel: [w357 w504] -> w348
                  frame False {
                    n211 = stacked-sequence {
                      seq-local: [w379 _ _] -> [_ w409 _]
                      seq-local: [w374 _ _] -> [_ _ w469]
                      seq-local: [w373 _ _] -> [_ _ w470]
                      tunnel: w361 -> [_ _ w475]
                      tunnel: w362 -> [_ _ w467]
                      tunnel: [_ _ w473] -> w364
                      tunnel: [_ _ w472] -> w360
                      tunnel: w363 -> [_ _ _]
                      tunnel: [w383 _ _] -> w359
                      tunnel: w358 -> [_ _ w461]
                      tunnel: [_ _ w460] -> w357
                      frame #0 {
                        w377 = T3."Add Element" ("Action")
                        # "SMU data"
                        n212 = Get Date/Time String(want seconds? (F)=TRUE) -> (time string=w380:string)  [unwired: 2 in, 1 out]
                        n213 = local write "Last reading at:"(w380) -> ()
                        n214 = local write "STATUS 1"("Reading current ..." ("status")) -> ()
                        n215 = global read "QC_MeasurementSetup.vi" "IV Measurement Parameters"() -> (w372:T8)
                        n216 = Unbundle By Name(w372) -> ("Supply"=w366:refnum<class "SupplyControl.lvclass">, "Set Current Limit?"=w371:bool, "Current Limit [µA]"=w368:dbl, "Temperature Readout"=w370:enum16{"Read Arduino", "Enter manually"}, "Arduino"=w365:refnum<class "ArduinoControl.lvclass">)
                        n217 = local read "Current reading No."() -> (w376:u32)
                        n218 = local read "Current Volts:"() -> (w385:dbl)
                        n219 = case shown="\"Read Arduino\"" w370 {
                          tunnel: [w393 w399] -> w381
                          tunnel: [w390 w398] -> w375
                          tunnel: w365 -> [_ w397]
                          frame "Enter manually", Default {
                            n220 = local read "Temp."() -> (w395:dbl[])
                            n221 = local read "RH"() -> (w391:dbl[])
                            n222 = Index Array(array=w395, index=0) -> (element=w393:dbl)
                            n223 = Index Array(array=w391, index=0) -> (element=w390:dbl)
                          }
                          frame "Read Arduino" {
                            n224 = call "ArduinoRead.vi"("Arduino function"=enum16{"T/RH", "Interlock", "Edgesense"}."T/RH", "ArduinoControl in"=w397) -> ("rel. Humidity [%]"=w398:dbl, "Temperature [°C]"=w399:dbl)  [unwired: 4 in, 4 out]
                          }
                        }
                        n225 = Multiply(x=w368, y=1000.0) -> (x*y=w367:dbl)
                        n226 = call-dynamic "Supply_ReadCurrent.vi"("SupplyControl in"=w366) -> ("error out"=w373:errorcluster, "Current in nA"=w384:dbl, "SupplyControl out"=w374:refnum<class "SupplyControl.lvclass">)  [unwired: 8 in]
                        n227 = case shown="True" w371 {
                          tunnel: w384 -> [_ w404]
                          tunnel: w367 -> [_ w402]
                          tunnel: [FALSE w401] -> w383
                          frame False {
                          }
                          frame True {
                            n228 = Absolute Value(x=w404) -> (abs(x)=w403:dbl)
                            n229 = Greater?(x=w403, y=w402) -> (0:w401:bool)
                          }
                        }
                        n230 = Increment(x=w376) -> (x+1=w379:u32)
                        n231 = call "IVData.vi"("Action"=w377, "Array No."=u32 1, "Data IN"=w384) -> ()  [unwired: 2 in, 2 out]
                        n232 = call "IVData.vi"("Action"=w377, "Array No."=0, "Data IN"=w385) -> ()  [unwired: 2 in, 2 out]
                        n233 = local write "Current reading No."(w379) -> ()
                        n234 = call "IVData.vi"("Action"=w377, "Array No."=u32 2, "Data IN"=w381) -> ()  [unwired: 2 in, 2 out]
                        n235 = call "IVData.vi"("Action"=w377, "Array No."=u32 3, "Data IN"=w375) -> ()  [unwired: 2 in, 2 out]
                      }
                      frame #1 {
                        w407 = T3."Read Array" ("Action")
                        w419 = u32 5 ("y")
                        # "Update plots"
                        n236 = property on="Igraph" class="XYGraph (strict)"() -> ("YScale.Mapping Mode"=w410:u8)  [unwired: 2 in, 2 out]
                        n237 = property on="Igraph" class="XYGraph (strict)"("YScale.Minimum"=w410) -> ()  [unwired: 2 in, 2 out]
                        n238 = call "IVData.vi"("Action"=w407, "Array No."=1) -> ("Array OUT"=w421:dbl[])  [unwired: 3 in, 1 out]
                        n239 = Greater?(x=w409, y=w419) -> (0:w418:bool)
                        n240 = case shown="False" w418 {
                          tunnel: w409 -> [w425 w428]
                          tunnel: w419 -> [_ w427]
                          tunnel: [w425 w427] -> w417
                          tunnel: [0 w426] -> w415
                          frame False {
                          }
                          frame True {
                            n241 = Subtract(x=w428, y=w427) -> (x-y=w426:u32)
                          }
                        }
                        n242 = Array Subset(array=w421, index=0, length=w409) -> (w414:dbl[])
                        n243 = local read "Iscale"() -> (w420:enum16{"nanoAmps", "microAmps", "milliAmps"})
                        n244 = Absolute Value(x=w414) -> (abs(x)=w413:dbl[])
                        n245 = case shown="..\"nanoAmps\"" w420 {
                          tunnel: [w453 w454 w457] -> w423
                          tunnel: w413 -> [w453 w456 w459]
                          frame .."nanoAmps" {
                          }
                          frame "microAmps" {
                            n246 = Divide(x=w456, y=1000.0) -> (x/y=w454:dbl[])
                          }
                          frame "milliAmps".. {
                            n247 = Divide(x=w459, y=1000000.0) -> (x/y=w457:dbl[])
                          }
                        }
                        n248 = call "IVData.vi"("Action"=w407, "Array No."=0) -> ("Array OUT"=w406:dbl[])  [unwired: 3 in, 1 out]
                        n249 = for {
                          N: 4 -> [_]
                          tunnel: w417 -> [w433]
                          tunnel: w415 -> [w432]
                          tunnel: w409 -> [w429]
                          i -> [w434]
                          n250 = call "IVData.vi"("Action"=T3."Read Array", "Array No."=w434) -> ("Array OUT"=w431:dbl[])  [unwired: 3 in, 1 out]
                          n251 = case shown="2" w434 {
                            tunnel: w433 -> [w437 w441 _ _]
                            tunnel: w432 -> [w438 w442 _ _]
                            tunnel: w431 -> [w436 w440 w446 w451]
                            tunnel: w429 -> [_ _ w444 w449]
                            frame ..0 {
                              n252 = Array Subset(array=w436, index=w438, length=w437) -> (w435:dbl[])
                              n253 = local write "Volts"(w435) -> ()
                            }
                            frame 1 {
                              n254 = Array Subset(array=w440, index=w442, length=w441) -> (w439:dbl[])
                              n255 = local write "Current"(w439) -> ()
                            }
                            frame 2 {
                              n256 = Decrement(x=w444) -> (x-1=w443:u32)
                              n257 = Array Subset(array=w446, index=w443, length=1) -> (w445:dbl[])
                              n258 = local write "Temp."(w445) -> ()
                            }
                            frame 3.. {
                              n259 = Decrement(x=w449) -> (x-1=w448:u32)
                              n260 = Array Subset(array=w451, index=w448, length=1) -> (w450:dbl[])
                              n261 = local write "RH"(w450) -> ()
                            }
                          }
                        }
                        n262 = Absolute Value(x=w406) -> (abs(x)=w405:dbl[])
                        n263 = Bundle(w405, w423) -> (w411:cluster{dbl[], dbl[]})  [unwired: 1 in]
                        n264 = local write "Igraph"(w411) -> ()
                      }
                      frame #2 {
                        # "Increment volts and check for end of loop"
                        n265 = local read "positive ramp?"() -> (w471:bool)
                        n266 = local read "Current Volts:"() -> (w462:dbl)
                        n267 = case shown="True" w471 {
                          tunnel: w467 -> [w478 w482]
                          tunnel: w475 -> [w479 w485]
                          tunnel: [w477 w484] -> w463
                          tunnel: [w476 w481] -> w474
                          tunnel: w462 -> [w480 w483]
                          frame False {
                            n268 = Subtract(x=w480, y=w479) -> (x-y=w476:dbl)
                            n269 = Greater Or Equal?(x=w476, y=w478) -> (x >= y?=w477:bool)
                          }
                          frame True {
                            n270 = Add(x=w483, y=w485) -> (x+y=w481:dbl)
                            n271 = Less Or Equal?(x=w481, y=w482) -> (x <= y?=w484:bool)
                          }
                        }
                        n272 = Quotient & Remainder(x=w462, y=w467) -> (x-y*floor(x/y)=w468:dbl, floor(x/y)=w466:dbl)
                        n273 = Not Equal To 0?(x=w468) -> (x != 0?=w464:bool)
                        n274 = Equal To 0?(x=w466) -> (x = 0?=w465:bool)
                        n275 = Or(x=w464, y=w465) -> ()  [unwired: 1 out]
                        n276 = case shown="True" w463 {
                          tunnel: w474 -> [_ w500]
                          tunnel: [w489 FALSE] -> w473
                          tunnel: [FALSE w501] -> w472
                          tunnel: w462 -> [_ w498]
                          tunnel: w470 -> [_ w497]
                          tunnel: w469 -> [_ w496]
                          tunnel: w461 -> [w488 _]
                          tunnel: [w487 0] -> w460
                          frame False {
                            (unwired) TRUE
                            n277 = Increment(x=w488) -> (x+1=w487:i32)
                            n278 = local read "hold steps"() -> (w486:i32)
                            n279 = Greater Or Equal?(x=w488, y=w486) -> (x >= y?=w489:bool)
                          }
                          frame True {
                            n280 = local read "step [V]"() -> (w494:dbl)
                            n281 = call "SupplyRamp.vi"("error in"=w497, "Requested Voltage"=w500, "Step Size"=w494, "Step Delay"=100, "Supply IN"=w496, "Starting Voltage"=w498) -> ("error out"=w492:errorcluster, "Compliance exceeded"=w501:bool, "Current Voltage"=w495:dbl)  [unwired: 2 in, 1 out]
                            n282 = local write "STATUS 1"("Incrementing volts.") -> ()
                            n283 = case shown="No Error" w492 {
                              tunnel: w495 -> [w503 _]
                              frame No Error {
                                n284 = local write "Current Volts:"(w503) -> ()
                              }
                              frame Error {
                              }
                            }
                            n285 = property on="Bias On/Off:" class="Bool (strict)"("Blinking"=w501) -> ()  [unwired: 2 in, 2 out]
                          }
                        }
                      }
                    }
                  }
                  frame True {
                    w505 = FALSE
                  }
                }
              }
            }
            n286 = case shown="True" w268 {
              frame False {
              }
              frame True {
                n287 = property on="Bias On/Off:" class="Bool (strict)"("Blinking"=TRUE) -> ()  [unwired: 2 in, 2 out]
              }
            }
            n288 = Build Array(w269, w268, "abort", w264) -> (w273:bool[])
            n289 = Or Array Elements(Boolean array=w273) -> (logical OR=w279:bool)
            n290 = Not(x=w279) -> (.not. x?=w278:bool)
          }
        }
        frame True {
          w507 = FALSE
          # "compliance was exceeded when first voltage applied."
          # "Flag compliance as reason for end of run"
          n291 = local write "STATUS 1"("Run aborted - compliance exceeded.") -> ()
          n292 = Build Array(w507, TRUE, w507, w507) -> (w508:bool[])
        }
      }
      n293 = Search 1D Array(1D array=w253, element=TRUE) -> (index of element=w251:i32)  [unwired: 1 in]
      n294 = Increment(x=w251) -> (x+1=w250:i32)
      n295 = case shown="2" w250 {
        tunnel: ["" "Run ended normally" "Compliance exceeded" "Run aborted - by user" "Run aborted - Ilimit exceeded"] -> w245
        frame ..0 {
        }
        frame 1 {
        }
        frame 2 {
          # "Determine reason for end of run."
        }
        frame 3 {
        }
        frame 4.. {
        }
      }
      n296 = global read "QC_RunInformation.vi" "Run info"() -> (w249:T7)
      n297 = Bundle By Name(cluster=w249, "End of Run comment:"=w245) -> (w244:T7)
      n298 = global write "QC_RunInformation.vi" "Run info"(w244) -> ()
      n299 = Concatenate Strings(w245, "\r\n", "RAMPING DOWN VOLTS") -> (w248:string)
      n300 = local write "STATUS 1"(w248) -> ()
    }
    frame #4 {
      # "Ramp down and switch off supply"
      n301 = stacked-sequence {
        frame #0 {
          # "Tie up loose ends. Set volts to zero and switch to standby"
          # "Ramp down volts now"
          n302 = global read "QC_MeasurementSetup.vi" "IV Measurement Parameters"() -> (w519:T8)
          n303 = Unbundle By Name(w519) -> ("Supply"=w516:refnum<class "SupplyControl.lvclass">, "Ramp down steps [V]"=w518:dbl, "Ramp down Interval [s]"=w517:i32, "Measurement switch"=w511:refnum<class "Switching.lvclass">, "Measurement switch used?"=w512:bool)
          n304 = Multiply(x=w517, y=1000) -> (x*y=w521:i32)
          n305 = local read "Current Volts:"() -> (w524:dbl)
          n306 = call "SupplyRamp.vi"("Requested Voltage"=0.0, "Step Size"=w518, "Step Delay"=w521, "Supply IN"=w516, "Starting Voltage"=w524) -> ("error out"=w515:errorcluster, "Supply OUT"=w514:refnum<class "SupplyControl.lvclass">, "Current Voltage"=w522:dbl)  [unwired: 3 in, 1 out]
          n307 = local write "Current Volts:"(w522) -> ()
          n308 = call-dynamic "Supply_Stby.vi"("error in (no error)"=w515, "SupplyControl in"=w514) -> ("error out"=w513:errorcluster)  [unwired: 8 in, 1 out]
          n309 = case shown="True" w512 {
            tunnel: w511 -> [_ w527]
            tunnel: w513 -> [_ w526]
            frame False {
            }
            frame True {
              n310 = call-dynamic "MatrixSwitch.vi"("error in (no error)"=w526, "Action"=T4."Reset", "Switching in"=w527) -> ()  [unwired: 6 in, 3 out]
            }
          }
        }
        frame #1 {
          w532 = 0
          n311 = local write "Bias On/Off:"(FALSE ("Visible")) -> ()
          n312 = local write "Current Volts:"(0.0 ("Current Volts:")) -> ()
          n313 = property on="Quit & Save" class="Bool"("DisabledEnum"=w532) -> ()  [unwired: 2 in, 2 out]
          n314 = property on="quit (no save)" class="Bool"("DisabledEnum"=w532) -> ()  [unwired: 2 in, 2 out]
          n315 = property on="abort" class="Bool (strict)"("DisabledEnum"=2) -> ()  [unwired: 2 in, 2 out]
          n316 = local write "STATUS 1"("Run finished. \nSave data?" ("STATUS 1")) -> ()
        }
        frame #2 {
          n317 = Current VI's Path() -> (path=w534:path)
          n318 = call "SaveJPEG.vi"("Test"="IV", "File Path Control"=w534) -> ()  [unwired: 1 in, 2 out]
        }
      }
    }
    frame #5 {
      # "Loop and await decision on whether to save or junk data"
      # "Display and save data"
      n319 = local read "Scales"() -> (w546:T1)
      n320 = local read "Iscale"() -> (w545:enum16{"nanoAmps", "microAmps", "milliAmps"})
      n321 = while {
        shift-left: w545 -> [w594]
        shift-right: [w593] -> _
        shift-left: w546 -> [w596]
        shift-right: [w595] -> _
        tunnel: ["Quit & Save"] -> w548
        tunnel: ["quit (no save)"] -> w547
        stop <- w591 continue-if-true
        n322 = local read "Scales"() -> (w595:T1)
        n323 = local read "Iscale"() -> (w593:enum16{"nanoAmps", "microAmps", "milliAmps"})
        n324 = Not Equal?(x=w596, y=w595) -> (x != y?=w589:bool)
        n325 = Not Equal?(x=w594, y=w593) -> (x != y?=w588:bool)
        n326 = case shown="True" w589 {
          tunnel: w595 -> [_ w623]
          frame False {
          }
          frame True {
            n327 = case shown="..\"Lin - Lin\"" w623 {
              tunnel: [w624 1 0 w629] -> w622
              tunnel: [w624 0 1 w629] -> w621
              frame .."Lin - Lin" {
                w624 = 0
              }
              frame "Log - Lin" {
              }
              frame "Lin - Log" {
              }
              frame "Log - log".. {
                w629 = 1
              }
            }
            n328 = property on="Igraph" class="XYGraph (strict)"("X Scale.Mapping Mode"=w622) -> ()  [unwired: 2 in, 2 out]
            n329 = property on="Igraph" class="XYGraph (strict)"("Y Scale.Mapping Mode"=w621, "YScale.Minimum"=w621) -> ()  [unwired: 2 in, 2 out]
          }
        }
        n330 = case shown="True" w588 {
          tunnel: w593 -> [_ w609]
          frame False {
          }
          frame True {
            w602 = T3."Read Array" ("Action")
            n331 = property on="Igraph" class="XYGraph (strict)"() -> ("YScale.Mapping Mode"=w605:u8)  [unwired: 2 in, 2 out]
            n332 = global read "QC_MeasurementSetup.vi" "IV Measurement Parameters"() -> (w604:T8)
            n333 = property on="Igraph" class="XYGraph (strict)"("YScale.Minimum"=w605) -> ()  [unwired: 2 in, 2 out]
            n334 = Unbundle By Name(w604) -> ("Number Of Steps"=w601:u32)
            n335 = local read "hold steps"() -> (w600:i32)
            n336 = Add(x=w601, y=w600) -> (x+y=w599:u32)
            n337 = call "IVData.vi"("Action"=w602, "Array No."=u32 1 ("Action")) -> ("Array OUT"=w611:dbl[])  [unwired: 3 in, 1 out]
            n338 = Array Subset(array=w611, index=0, length=w599) -> (w608:dbl[])
            n339 = Absolute Value(x=w608) -> (abs(x)=w607:dbl[])
            n340 = case shown="\"microAmps\"" w609 {
              tunnel: [w614 w615 w619] -> w613
              tunnel: w607 -> [w614 w617 w620]
              frame .."nanoAmps" {
              }
              frame "microAmps" {
                n341 = Divide(x=w617, y=1000.0) -> (x/y=w615:dbl[])
              }
              frame "milliAmps".. {
                n342 = Divide(x=w620, y=1000000.0) -> (x/y=w619:dbl[])
              }
            }
            n343 = call "IVData.vi"("Action"=w602, "Array No."=u32 0 ("Action")) -> ("Array OUT"=w598:dbl[])  [unwired: 3 in, 1 out]
            n344 = Absolute Value(x=w598) -> (abs(x)=w597:dbl[])
            n345 = Bundle(w597, w613) -> (w610:cluster{dbl[], dbl[]})  [unwired: 1 in]
            n346 = local write "Igraph"(w610) -> ()
          }
        }
        n347 = local read "Run uninterrupted?"() -> (w587:bool)
        n348 = Compound Arithmetic op=OR("Quit & Save", "quit (no save)", w587) -> (invert w591:bool)
      }
      n349 = global read "QC_MeasurementSetup.vi" "IV Measurement Parameters"() -> (w544:T8)
      n350 = Unbundle By Name(w544) -> ("Temperature Readout"=w543:enum16{"Read Arduino", "Enter manually"}, "Arduino"=w537:refnum<class "ArduinoControl.lvclass">)
      n351 = case shown="\"Read Arduino\"" w543 {
        tunnel: w537 -> [_ w586]
        frame "Enter manually", Default {
        }
        frame "Read Arduino" {
          n352 = call "ArduinoClose.vi"("ArduinoControl in"=w586) -> ()  [unwired: 9 in, 2 out]
        }
      }
      n353 = case shown="True" w547 {
        tunnel: [FALSE w631] -> w549
        frame False {
        }
        frame True {
          n354 = Two Button Dialog(message="Are you sure you don't want to save the data?", 1:"Quit" ("F button name (\"Cancel\")"), 2:"Save data" ("T button name (\"OK\")")) -> (T button?=w631:bool)
        }
      }
      n355 = local read "Run uninterrupted?"() -> (w535:bool)
      n356 = Compound Arithmetic op=OR(w548, w549, w535) -> (w542:bool)
      n357 = flat-sequence {
        tunnel: w542 -> [w552]
        tunnel: [w552] -> w538
        tunnel: [TRUE] -> w536
        tunnel: w535 -> [w550]
        frame #0 {
          n358 = global read "QC_MeasurementSetup.vi" "IV Measurement Parameters"() -> (w562:T8)
          n359 = Unbundle By Name(w562) -> ("V_breakdown Limit [V]"=w556:dbl, "Number Of Steps"=w557:u32)
          n360 = call "ScanFeedback.vi"("measurement type"=T5."IV") -> ("V breakdown"=w554:dbl)  [unwired: 4 in, 4 out]
          n361 = Absolute Value(x=w554) -> (abs(x)=w553:dbl)
          n362 = Absolute Value(x=w556) -> (abs(x)=w555:dbl)
          n363 = case shown="True" w552 {
            tunnel: ["" w585] -> w563
            tunnel: [_ w571] -> w561
            tunnel: w557 -> [_ w569]
            tunnel: w550 -> [_ w566]
            frame False {
            }
            frame True {
              w581 = T3."Read Array" ("Action")
              n364 = local read "hold steps"() -> (w568:i32)
              n365 = Add(x=w569, y=w568) -> ()  [unwired: 1 out]
              n366 = local write "STATUS 1"("Saving Data ...") -> ()
              n367 = call "IVData.vi"("Action"=w581, "Array No."=u32 0 ("Action")) -> ("Array OUT"=w565:dbl[])  [unwired: 3 in, 1 out]
              n368 = call "IVData.vi"("Action"=w581, "Array No."=u32 1 ("Action")) -> ("Array OUT"=w576:dbl[])  [unwired: 3 in, 1 out]
              n369 = call "IVData.vi"("Action"=w581, "Array No."=u32 3 ("Action")) -> ("Array OUT"=w583:dbl[])  [unwired: 3 in, 1 out]
              n370 = call "IVData.vi"("Action"=w581, "Array No."=u32 2 ("Action")) -> ("Array OUT"=w582:dbl[])  [unwired: 3 in, 1 out]
              n371 = call <vilib>:"Std Deviation and Variance.vi"("X"=w583) -> ("mean"=w572:dbl)  [unwired: 1 in, 2 out]
              n372 = call <vilib>:"Std Deviation and Variance.vi"("X"=w582) -> ("mean"=w573:dbl)  [unwired: 1 in, 2 out]
              n373 = Build Array(w565, w576) -> (w575:dbl[][])
              n374 = Transpose 2D Array(2D array=w575) -> ()  [unwired: 1 out]
              n375 = call "SaveDataFile.vi"("Temperature"=w573, "Run uninterrupted?"=w566, "Humidity"=w572, "Array Titles"="Voltage[V] Current[nA]", "Strip Segment"="", "Arrays format"="%010.2f") -> ("Path + Filename OUT"=w585:string, "Error Out"=w571:errorcluster)  [unwired: 6 in, 2 out]
            }
          }
          n376 = Greater Or Equal?(x=w553, y=w555) -> (x >= y?=w558:bool)
          n377 = call "WriteLogFile.vi"("Run uninterrupted?"=w550, "Automatic warning"="", "Data File"=w563, "Error In"=w561, "DUT passed?"=w558, "Value TechSpec criteria"=w554, "Files saved?"=w552) -> ()  [unwired: 4 in, 1 out]
        }
      }
      n378 = Select(t="Run finished.\nData saved." ("STATUS 1"), s=w538, f="Run finished.\nData not saved." ("STATUS 1")) -> (s? t:f=w541:string)
      n379 = local write "STATUS 1"(w541) -> ()
      "Done!" <- w536
    }
  }
